vi "G2CPU Create Line Profile Indexers.vi"(6 "Auto Release Line Points":T2={"Auto Release Points 1 X (enabled)"=TRUE, "Auto Release Points 1 Y (enabled)"=TRUE, "Auto Release Points 2 X (enabled)"=TRUE, "Auto Release Points 2 Y (enabled)"=TRUE, "Auto Release Keys (enabled)"=TRUE}, 8 "error in (no error)":errorcluster, 10 "Lines":T3, 11 "Greyscale Image In":refnum<class "2D Array f32.lvclass">) -> (0 "error out":errorcluster, 2 "Line Indexers":T1, 3 "Greyscale Image Out (inplace)":refnum<class "2D Array f32.lvclass">)   [LabVIEW 2020, in "G2CPU Line Profile.lvlib"]
doc: "Create a set of flattened indexes representing the coordinates of each pixel in a line profile."
uses:
  G2CPU Line Profile.lvlib
  <vilib>/Natan Biesmans/G2CPU GPU and CPU HPC Toolkit/G2CPU Libraries/Arrays/2DArray/f32/2D Array f32.lvclass
  C:/Program Files/National Instruments/LabVIEW 2025/vi.lib/Natan Biesmans/G2CPU GPU and CPU HPC Toolkit/G2CPU Libraries/Arrays/Array/Array Prototype.lvclass
  <vilib>/Natan Biesmans/G2CPU GPU and CPU HPC Toolkit/G2CPU Libraries/Arrays/1DArray/f32/1D Array f32.lvclass
  <vilib>/Natan Biesmans/G2CPU GPU and CPU HPC Toolkit/G2CPU Libraries/Arrays/1DArray/u32/1D Array u32.lvclass
  <vilib>/Natan Biesmans/G2CPU GPU and CPU HPC Toolkit/G2CPU Libraries/Arrays/2DArray/u32/2D Array u32.lvclass
  <vilib>/Natan Biesmans/G2CPU GPU and CPU HPC Toolkit/G2CPU Libraries/Arrays/Array/Array Prototype.lvclass/Array Prototype.ctl
  b2d675fe-ffa8-47e0-b07b-14ad1d69e3ae.vi
  068896be-3049-4794-95f3-18267501b1a4.vi
  474dc051-b38d-4f18-9454-ae451d7f23ba.vi
  598d86ab-c10d-4ab8-84aa-0b74b9baac51.vi
  789355b7-c740-4406-be93-379218f93cff.vi
  e515b795-e06e-4ce0-815c-d9762167fd43.vi
  f1fa9f08-163f-4c38-a6b5-bfbcbea63e99.vi
  e5122186-ef43-49a6-80ad-7344628695c2.vi
  09d3c97f-016e-4235-b4d3-386cf7d802b8.vi
  743f27c3-c532-4a2e-9500-26ef6d7e19b8.vi
  018279aa-aab3-48a4-bb93-401516e76ec1.vi
  5bbf4c43-7f87-459e-811e-5969f3ec3ecc.vi
  502ba427-d302-48ff-a4ea-f7cba77dd3ea.vi
  <vilib>/Natan Biesmans/G2CPU GPU and CPU HPC Toolkit/G2CPU Libraries/Arrays/Array/G2CPU Get Array Pointer.vi
  b2d675fe-ffa8-47e0-b07b-14ad1d69e3ae.vi/4181b2af-0669-475f-8228-b34a8d51a6f4.vi
  068896be-3049-4794-95f3-18267501b1a4.vi/4181b2af-0669-475f-8228-b34a8d51a6f4.vi
  474dc051-b38d-4f18-9454-ae451d7f23ba.vi/4181b2af-0669-475f-8228-b34a8d51a6f4.vi
  598d86ab-c10d-4ab8-84aa-0b74b9baac51.vi/4181b2af-0669-475f-8228-b34a8d51a6f4.vi
  789355b7-c740-4406-be93-379218f93cff.vi/46771f49-eb1d-473b-8e81-f516cef50a4e.vi
  789355b7-c740-4406-be93-379218f93cff.vi/dc76f8e4-64fa-456a-8549-7a4b6936c4c9.vi
  789355b7-c740-4406-be93-379218f93cff.vi/7e60ddfb-e748-4c0c-85da-e395a1b7978d.vi
  789355b7-c740-4406-be93-379218f93cff.vi/d2eceff7-f641-4ce4-acfa-e9e293a3c877.vi
  789355b7-c740-4406-be93-379218f93cff.vi/b737122b-4036-448b-abd3-e2701355e828.vi
  e515b795-e06e-4ce0-815c-d9762167fd43.vi/d8f9d983-4edf-44a2-8364-f00f0b470774.vi
  e515b795-e06e-4ce0-815c-d9762167fd43.vi/83167447-a0f5-45d9-a71d-4def8f50970d.vi
  f1fa9f08-163f-4c38-a6b5-bfbcbea63e99.vi/4181b2af-0669-475f-8228-b34a8d51a6f4.vi
  e5122186-ef43-49a6-80ad-7344628695c2.vi/1bf6e03b-eb75-45f6-9764-49dc38a3a024.vi
  e5122186-ef43-49a6-80ad-7344628695c2.vi/2da4419f-02df-47a7-be00-1b7e0871fa33.vi
  09d3c97f-016e-4235-b4d3-386cf7d802b8.vi/80f98885-d133-4778-8a71-11569f5a634e.vi
  09d3c97f-016e-4235-b4d3-386cf7d802b8.vi/fede99c7-5d82-4ae2-b666-3731d213e31f.vi
  743f27c3-c532-4a2e-9500-26ef6d7e19b8.vi/cfed8f62-9c64-4dab-912e-5e7c21cb720b.vi
  018279aa-aab3-48a4-bb93-401516e76ec1.vi/d8f9d983-4edf-44a2-8364-f00f0b470774.vi
  018279aa-aab3-48a4-bb93-401516e76ec1.vi/83167447-a0f5-45d9-a71d-4def8f50970d.vi
  5bbf4c43-7f87-459e-811e-5969f3ec3ecc.vi/cfed8f62-9c64-4dab-912e-5e7c21cb720b.vi
  502ba427-d302-48ff-a4ea-f7cba77dd3ea.vi/5793b77b-c002-4ebf-9075-685617c95341.vi
  502ba427-d302-48ff-a4ea-f7cba77dd3ea.vi/2ed3ef86-c00d-4d71-b84c-20267a6dfcf9.vi
  789355b7-c740-4406-be93-379218f93cff.vi/dc76f8e4-64fa-456a-8549-7a4b6936c4c9.vi/3e802c67-fb96-46a3-ae13-4994a8508b4f.vi
  789355b7-c740-4406-be93-379218f93cff.vi/dc76f8e4-64fa-456a-8549-7a4b6936c4c9.vi/5a50fc67-79e7-4972-80c2-92243cd53dd4.vi
  789355b7-c740-4406-be93-379218f93cff.vi/dc76f8e4-64fa-456a-8549-7a4b6936c4c9.vi/1c928fc9-710a-40e7-8c4f-08a1069452ae.vi
  e5122186-ef43-49a6-80ad-7344628695c2.vi/1bf6e03b-eb75-45f6-9764-49dc38a3a024.vi/3e802c67-fb96-46a3-ae13-4994a8508b4f.vi
  e5122186-ef43-49a6-80ad-7344628695c2.vi/1bf6e03b-eb75-45f6-9764-49dc38a3a024.vi/5a50fc67-79e7-4972-80c2-92243cd53dd4.vi
  e5122186-ef43-49a6-80ad-7344628695c2.vi/2da4419f-02df-47a7-be00-1b7e0871fa33.vi/730f6c57-5c0b-4ee9-b61e-75067b25222b.vi
  e5122186-ef43-49a6-80ad-7344628695c2.vi/2da4419f-02df-47a7-be00-1b7e0871fa33.vi/096b8799-7810-404e-baca-ba9279cec4bd.vi
  e5122186-ef43-49a6-80ad-7344628695c2.vi/2da4419f-02df-47a7-be00-1b7e0871fa33.vi/0f1a5a47-bcc5-4796-ac31-8dfcfbc0d7d1.vi
  e5122186-ef43-49a6-80ad-7344628695c2.vi/2da4419f-02df-47a7-be00-1b7e0871fa33.vi/89f12e17-3330-4b72-ad8f-8dd636660732.vi
  09d3c97f-016e-4235-b4d3-386cf7d802b8.vi/80f98885-d133-4778-8a71-11569f5a634e.vi/6058dca8-195d-4566-b47b-6d6a1c5af61f.vi
  743f27c3-c532-4a2e-9500-26ef6d7e19b8.vi/cfed8f62-9c64-4dab-912e-5e7c21cb720b.vi/77c7badc-ed81-4514-99c1-20d37f4e5ecc.vi
  743f27c3-c532-4a2e-9500-26ef6d7e19b8.vi/cfed8f62-9c64-4dab-912e-5e7c21cb720b.vi/eb76fa01-6782-47b4-b34f-9eb474c9cc78.vi
  <vilib>/Natan Biesmans/G2CPU GPU and CPU HPC Toolkit/ArrayFire Driver/VIs/Run as Multi Device.vi
  5bbf4c43-7f87-459e-811e-5969f3ec3ecc.vi/cfed8f62-9c64-4dab-912e-5e7c21cb720b.vi/77c7badc-ed81-4514-99c1-20d37f4e5ecc.vi
  5bbf4c43-7f87-459e-811e-5969f3ec3ecc.vi/cfed8f62-9c64-4dab-912e-5e7c21cb720b.vi/eb76fa01-6782-47b4-b34f-9eb474c9cc78.vi
  502ba427-d302-48ff-a4ea-f7cba77dd3ea.vi/5793b77b-c002-4ebf-9075-685617c95341.vi/3e802c67-fb96-46a3-ae13-4994a8508b4f.vi
  502ba427-d302-48ff-a4ea-f7cba77dd3ea.vi/5793b77b-c002-4ebf-9075-685617c95341.vi/5a50fc67-79e7-4972-80c2-92243cd53dd4.vi
  502ba427-d302-48ff-a4ea-f7cba77dd3ea.vi/2ed3ef86-c00d-4d71-b84c-20267a6dfcf9.vi/730f6c57-5c0b-4ee9-b61e-75067b25222b.vi
  502ba427-d302-48ff-a4ea-f7cba77dd3ea.vi/2ed3ef86-c00d-4d71-b84c-20267a6dfcf9.vi/096b8799-7810-404e-baca-ba9279cec4bd.vi
  502ba427-d302-48ff-a4ea-f7cba77dd3ea.vi/2ed3ef86-c00d-4d71-b84c-20267a6dfcf9.vi/0f1a5a47-bcc5-4796-ac31-8dfcfbc0d7d1.vi
  502ba427-d302-48ff-a4ea-f7cba77dd3ea.vi/2ed3ef86-c00d-4d71-b84c-20267a6dfcf9.vi/89f12e17-3330-4b72-ad8f-8dd636660732.vi
  789355b7-c740-4406-be93-379218f93cff.vi/dc76f8e4-64fa-456a-8549-7a4b6936c4c9.vi/3e802c67-fb96-46a3-ae13-4994a8508b4f.vi/1b7cf390-2ae0-48f3-9bce-03c57eed6ee8.vi
  09d3c97f-016e-4235-b4d3-386cf7d802b8.vi/80f98885-d133-4778-8a71-11569f5a634e.vi/6058dca8-195d-4566-b47b-6d6a1c5af61f.vi/77c7badc-ed81-4514-99c1-20d37f4e5ecc.vi
  09d3c97f-016e-4235-b4d3-386cf7d802b8.vi/80f98885-d133-4778-8a71-11569f5a634e.vi/6058dca8-195d-4566-b47b-6d6a1c5af61f.vi/eb76fa01-6782-47b4-b34f-9eb474c9cc78.vi
  502ba427-d302-48ff-a4ea-f7cba77dd3ea.vi/2ed3ef86-c00d-4d71-b84c-20267a6dfcf9.vi/730f6c57-5c0b-4ee9-b61e-75067b25222b.vi/0070e0fe-4ad7-4a3e-8965-d64becb7e5f0.vi
  <vilib>/Natan Biesmans/G2CPU GPU and CPU HPC Toolkit/G2CPU Libraries/Arrays/2DArray/binary/2D Array binary.lvclass
  <vilib>/Natan Biesmans/G2CPU GPU and CPU HPC Toolkit/ArrayFire Driver/VIs/round.vi
  <vilib>/Natan Biesmans/G2CPU GPU and CPU HPC Toolkit/G2CPU Libraries/Arrays/Array/G2CPU Set Array Pointer.vi
  <vilib>/Natan Biesmans/G2CPU GPU and CPU HPC Toolkit/ArrayFire Driver/subvi/Error Converter (ErrCode or Status).vi
  <vilib>/Natan Biesmans/G2CPU GPU and CPU HPC Toolkit/G2CPU Libraries/Arrays/SubVI/is 1D.vi
  <vilib>/Natan Biesmans/G2CPU GPU and CPU HPC Toolkit/ArrayFire Driver/VIs/div.vi
  <vilib>/Natan Biesmans/G2CPU GPU and CPU HPC Toolkit/ArrayFire Driver/VIs/replace.vi
  <vilib>/Natan Biesmans/G2CPU GPU and CPU HPC Toolkit/G2CPU Libraries/Arrays/SubVI/is 2D.vi
  <vilib>/Natan Biesmans/G2CPU GPU and CPU HPC Toolkit/ArrayFire Driver/VIs/sub.vi
  <vilib>/Natan Biesmans/G2CPU GPU and CPU HPC Toolkit/ArrayFire Driver/VIs/iszero.vi
  <vilib>/Natan Biesmans/G2CPU GPU and CPU HPC Toolkit/ArrayFire Driver/VIs/release array.vi
  <vilib>/Natan Biesmans/G2CPU GPU and CPU HPC Toolkit/ArrayFire Driver/VIs/cast.vi
  <vilib>/Natan Biesmans/G2CPU GPU and CPU HPC Toolkit/ArrayFire Driver/VIs/add.vi
  <vilib>/Natan Biesmans/G2CPU GPU and CPU HPC Toolkit/ArrayFire Driver/VIs/ge.vi
  <vilib>/Natan Biesmans/G2CPU GPU and CPU HPC Toolkit/G2CPU Libraries/Arrays/Array/Array Prototype.lvclass
  <vilib>/Natan Biesmans/G2CPU GPU and CPU HPC Toolkit/G2CPU Libraries/Arrays/DataTypes/f32/f32.lvclass
  <vilib>/Natan Biesmans/G2CPU GPU and CPU HPC Toolkit/G2CPU Libraries/Arrays/1DArray/1D Array Prototype.lvclass
  <vilib>/Natan Biesmans/G2CPU GPU and CPU HPC Toolkit/G2CPU Libraries/Arrays/2DArray/2D Array Prototype.lvclass
  <vilib>/Natan Biesmans/G2CPU GPU and CPU HPC Toolkit/G2CPU Libraries/Arrays/DataTypes/U32/U32.lvclass
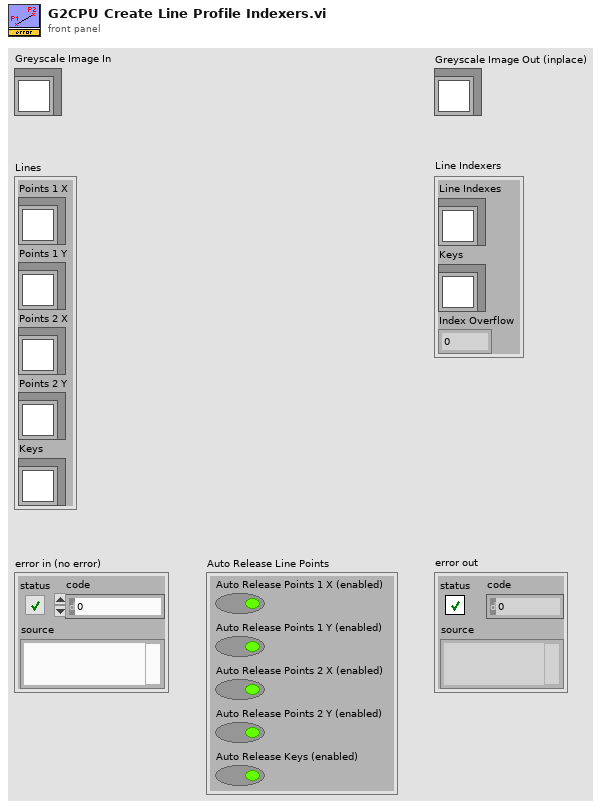
[diagram p1: front panel]
types:
  T1 = cluster{"Line Indexes":refnum<class "2D Array f32.lvclass">, "Keys":refnum<class "2D Array u32.lvclass">, "Index Overflow":u64}
  T2 = cluster{"Auto Release Points 1 X (enabled)":bool, "Auto Release Points 1 Y (enabled)":bool, "Auto Release Points 2 X (enabled)":bool, "Auto Release Points 2 Y (enabled)":bool, "Auto Release Keys (enabled)":bool}
  T3 = cluster{"Points 1 X":refnum<class "1D Array f32.lvclass">, "Points 1 Y":refnum<class "1D Array f32.lvclass">, "Points 2 X":refnum<class "1D Array f32.lvclass">, "Points 2 Y":refnum<class "1D Array f32.lvclass">, "Keys":refnum<class "1D Array u32.lvclass">}
  T4 = typedef "AF.lvlib/Dim4.ctl" = cluster{"Dim 0":u64, "Dim 1":u64, "Dim 2":u64, "Dim 3":u64}
  T5 = cluster{"Dim 0":sgl, "Dim 1":sgl, "Dim 2":sgl, "Dim 3":sgl}
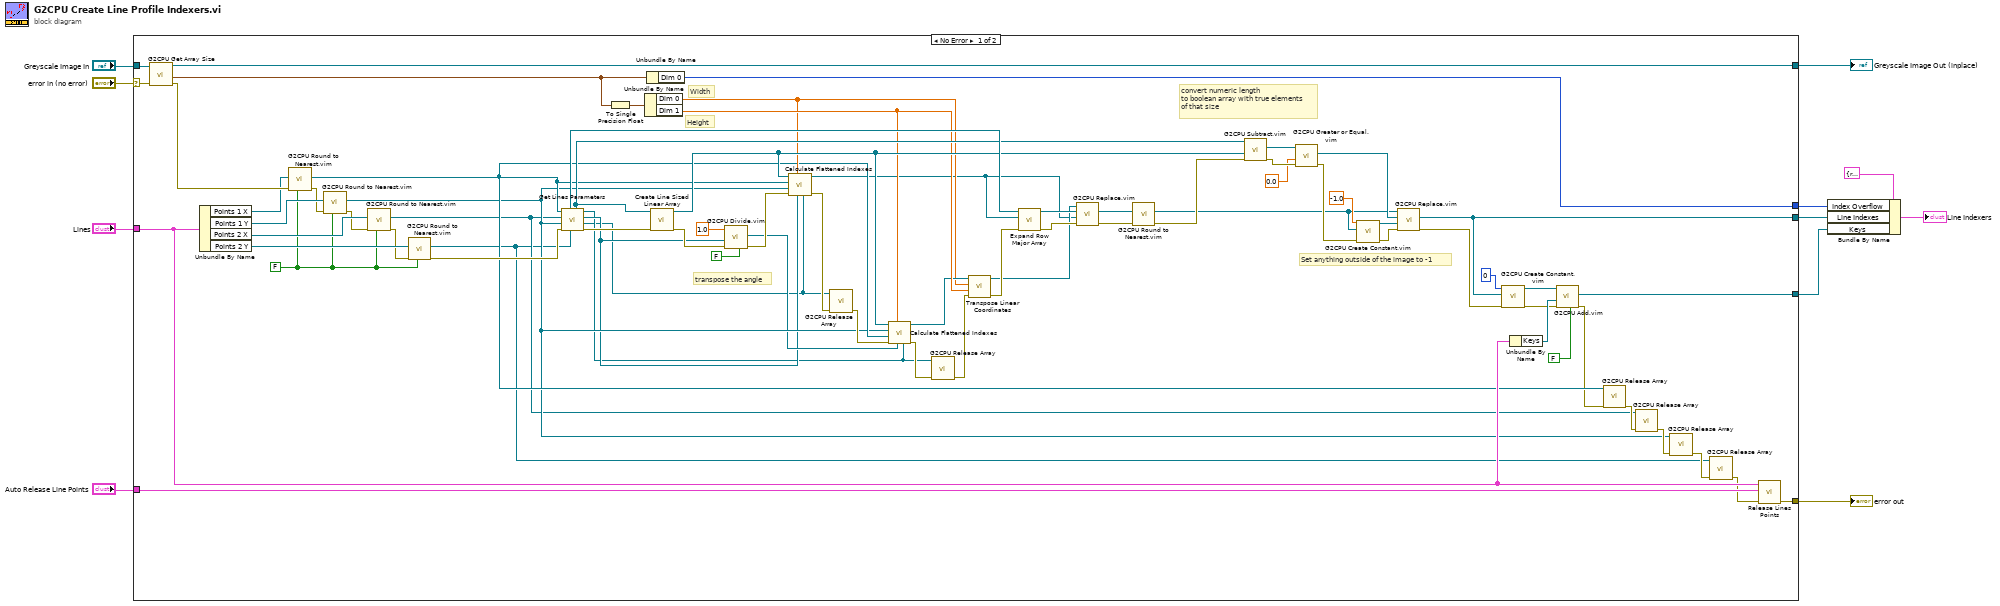
[diagram p0: block diagram]
diagram:
  n1 = case shown="No Error" "error in (no error)" {
    selector: "error in (no error)" -> [w82 w85]
    tunnel: "Greyscale Image In" -> [w83 w84]
    tunnel: "Lines" -> [w37 _]
    tunnel: [w51 _] -> w5
    tunnel: [w58 w84] -> w8
    tunnel: [w44 w85] -> w7
    tunnel: "Auto Release Line Points" -> [w57 _]
    tunnel: [w45 _] -> w4
    tunnel: [w42 _] -> w3
    frame No Error {
      w26 = FALSE ("Auto Release (Enabled)")
      # "Set anything outside of the image to -1"
      # "convert numeric length\nto boolean array with true elements\nof that size"
      # "transpose the angle"
      # "Height"
      # "Width"
      n2 = call <vilib>:"G2CPU Get Array Size.vi"("error in (no error)"=w82, "Array in"=w83) -> ("error out"=w39:errorcluster, "Array Size"=w43:T4, "Array out"=w58:refnum<class "2D Array f32.lvclass">)  [unwired: 6 in, 1 out]
      n3 = Unbundle By Name(w37) -> ("Points 1 X"=w33:refnum<class "1D Array f32.lvclass">, "Points 1 Y"=w32:refnum<class "1D Array f32.lvclass">, "Points 2 X"=w31:refnum<class "1D Array f32.lvclass">, "Points 2 Y"=w30:refnum<class "1D Array f32.lvclass">)
      n4 = call "G2CPU Round to Nearest.vim"("Auto Release (Enabled)"=w26, "error in (no error)"=w39, "Array in"=w33) -> ("error out"=w29:errorcluster, "Array Result"=w25:refnum<class "1D Array f32.lvclass">)  [unwired: 7 in]
      n5 = call "G2CPU Round to Nearest.vim"("Auto Release (Enabled)"=w26, "error in (no error)"=w29, "Array in"=w32) -> ("error out"=w28:errorcluster, "Array Result"=w24:refnum<class "1D Array f32.lvclass">)  [unwired: 7 in]
      n6 = call "G2CPU Round to Nearest.vim"("Auto Release (Enabled)"=w26, "error in (no error)"=w28, "Array in"=w31) -> ("error out"=w27:errorcluster, "Array Result"=w23:refnum<class "1D Array f32.lvclass">)  [unwired: 7 in]
      n7 = call "G2CPU Round to Nearest.vim"("Auto Release (Enabled)"=w26, "error in (no error)"=w27, "Array in"=w30) -> ("error out"=w38:errorcluster, "Array Result"=w22:refnum<class "1D Array f32.lvclass">)  [unwired: 7 in]
      n8 = call "Get Lines Parameters.vi"("P2 Y (unreleased)"=w22, "error in (no error)"=w38, "P1 Y (unreleased)"=w24, "P2 X (unreleased)"=w23, "P1 X (unreleased)"=w25) -> ("error out"=w59:errorcluster, "Quadrant Correction X"=w13:refnum<class "1D Array f32.lvclass">, "Direction Coefficients"=w15:refnum<class "1D Array f32.lvclass">, "Quadrant Correction Y"=w14:refnum<class "1D Array f32.lvclass">, "Length of Lines"=w71:refnum<class "1D Array f32.lvclass">, "Is Row Major Line"=w78:refnum<class "1D Array binary.lvclass">)  [unwired: 1 in]
      n9 = To Single Precision Float(number=w43) -> (single precision float=w64:T5)
      n10 = Unbundle By Name(w64) -> ("Dim 0"=w40:sgl, "Dim 1"=w63:sgl)
      n11 = Unbundle By Name(w43) -> ("Dim 0"=w42:u64)
      n12 = call "Create Line Sized Linear Array.vi"("error in (no error)"=w59, "Line Sizes (unreleased)"=w71) -> ("error out"=w69:errorcluster, "Line Sized Linear Array"=w72:refnum<class "2D Array f32.lvclass">)  [unwired: 7 in, 1 out]
      n13 = call "G2CPU Divide.vim"("Auto Release rhs (Enabled)"=FALSE, "error in (no error)"=w69, "Array rhs"=w15, "Array lhs"=sgl 1.0 ("Datatype")) -> ("error out"=w70:errorcluster, "Array Result"=w16:refnum<class "1D Array f32.lvclass">)  [unwired: 6 in]
      n14 = call "Calculate Flattened Indexes.vi"("Q2 Q3 modifier (unreleased)"=w13, "Angle"=w15, "Image Size"=w40, "error in (no error)"=w70, "Relative X (unreleased)"=w24, "Relative Y (unreleased)"=w25, "Range In (unreleased)"=w72) -> ("error out"=w80:errorcluster, "Range Out"=w17:refnum<class "2D Array f32.lvclass">)  [unwired: 3 in]
      n15 = call <vilib>:"G2CPU Release Array.vi"("error in (no error)"=w80, "Array in"=w13) -> ("error out"=w81:errorcluster)  [unwired: 9 in]
      n16 = call "Calculate Flattened Indexes.vi"("Q2 Q3 modifier (unreleased)"=w14, "Angle"=w16, "Image Size"=w63, "error in (no error)"=w81, "Relative X (unreleased)"=w25, "Relative Y (unreleased)"=w24, "Range In (unreleased)"=w72) -> ("error out"=w79:errorcluster, "Range Out"=w62:refnum<class "2D Array f32.lvclass">)  [unwired: 3 in]
      n17 = call <vilib>:"G2CPU Release Array.vi"("error in (no error)"=w79, "Array in"=w14) -> ("error out"=w21:errorcluster)  [unwired: 9 in]
      n18 = call "Transpose Linear Coordinates.vi"("error in (no error)"=w21, "Dim 1"=w63, "Dim 0"=w40, "Transposed Linear Coordinates"=w62) -> ("error out"=w68:errorcluster, "Corrected Linear Coordinates"=w18:refnum<class "2D Array f32.lvclass">)  [unwired: 6 in]
      n19 = call "Expand Row Major Array.vi"("Error in"=w68, "Output Size (unreleased)"=w17, "1D Row Major In"=w78) -> ("error out"=w77:errorcluster, "2D Row Major Out"=w65:refnum<class "2D Array binary.lvclass">)  [unwired: 7 in]
      n20 = call "G2CPU Replace.vim"("error in (no error)"=w77, "To Replace Values Array or scalar Value"=w17, "Replace  Condition"=w65, "Array In"=w18) -> ("error out"=w67:errorcluster, "Array out (same as in)"=w66:refnum<class "2D Array f32.lvclass">)  [unwired: 6 in]
      n21 = call "G2CPU Round to Nearest.vim"("error in (no error)"=w67, "Array in"=w66) -> ("error out"=w76:errorcluster, "Array Result"=w12:refnum<class "2D Array f32.lvclass">)  [unwired: 8 in]
      n22 = call "G2CPU Subtract.vim"("error in (no error)"=w76, "Array rhs"=w72, "Array lhs"=w71) -> ("error out"=w75:errorcluster, "Array Result"=w73:refnum<class "2D Array f32.lvclass">)  [unwired: 7 in]
      n23 = call "G2CPU Greater or Equal.vim"("error in (no error)"=w75, "Array rhs"=sgl 0.0 ("Datatype"), "Array lhs"=w73) -> ("error out"=w54:errorcluster, "Array Result"=w53:refnum<class "2D Array binary.lvclass">)  [unwired: 7 in]
      n24 = call "G2CPU Create Constant.vim"("error in (no error)"=w54, "Size"=w12, "val"=sgl -1.0 ("Datatype Prototype")) -> ("error out"=w55:errorcluster, "object out"=w56:refnum<class "2D Array f32.lvclass">)  [unwired: 7 in]
      n25 = call "G2CPU Replace.vim"("error in (no error)"=w55, "To Replace Values Array or scalar Value"=w56, "Replace  Condition"=w53, "Array In"=w12) -> ("error out"=w50:errorcluster, "Array out (same as in)"=w51:refnum<class "2D Array f32.lvclass">)  [unwired: 6 in]
      n26 = call "G2CPU Create Constant.vim"("error in (no error)"=w50, "Size"=w51, "val"=u32 0) -> ("error out"=w46:errorcluster, "object out"=w48:refnum<class "2D Array u32.lvclass">)  [unwired: 7 in]
      n27 = Unbundle By Name(w37) -> ("Keys"=w47:refnum<class "1D Array u32.lvclass">)
      n28 = call "G2CPU Add.vim"("Auto Release rhs (Enabled)"=FALSE, "error in (no error)"=w46, "Array rhs"=w47, "Array lhs"=w48) -> ("error out"=w20:errorcluster, "Array Result"=w45:refnum<class "2D Array u32.lvclass">)  [unwired: 6 in]
      n29 = call <vilib>:"G2CPU Release Array.vi"("error in (no error)"=w20, "Array in"=w25) -> ("error out"=w36:errorcluster)  [unwired: 9 in]
      n30 = call <vilib>:"G2CPU Release Array.vi"("error in (no error)"=w36, "Array in"=w23) -> ("error out"=w35:errorcluster)  [unwired: 9 in]
      n31 = call <vilib>:"G2CPU Release Array.vi"("error in (no error)"=w35, "Array in"=w24) -> ("error out"=w34:errorcluster)  [unwired: 9 in]
      n32 = call <vilib>:"G2CPU Release Array.vi"("error in (no error)"=w34, "Array in"=w22) -> ("error out"=w19:errorcluster)  [unwired: 9 in]
      n33 = call "Release Lines Points.vi"("error in (no error)"=w19, "Auto Release  Line Points"=w57, "Lines"=w37) -> ("error out"=w44:errorcluster)  [unwired: 8 in]
    }
    frame Error {
    }
  }
  "error out" <- w7
  "Greyscale Image Out (inplace)" <- w8
  n34 = Bundle By Name(cluster=T1 {"Line Indexes"=refnum, "Keys"=refnum, "Index Overflow"=0} ("Line Indexers"), "Index Overflow"=w3, "Line Indexes"=w5, "Keys"=w4) -> (→"Line Indexers":T1)
